vi "Rx Channel Section.vi"(8 "error in (no error)":errorcluster, 11 "Node Ptr":T1 format="%.0x") -> (0 "error out":errorcluster)   [LabVIEW 2019, in "UDP-Custom-Device System Explorer.lvlib"]
uses:
  UDP-Custom-Device System Explorer.lvlib
  <vilib>/NI VeriStand/Custom Device API/Custom Device Item Ref.ctl
  <vilib>/NI VeriStand/Custom Device API/Custom Device API.lvlib
panel:
  in  "Description":string
  out "Name":string
  in  "SHDocVw.IWebBrowser":refnum<k7>(container)
  in  "General Header":cluster{"Section Name":string}={"Section Name"="Receive Channels"}
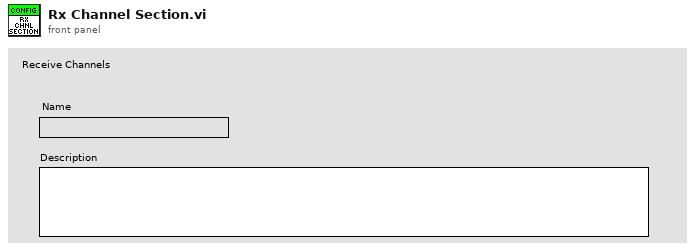
[diagram p1: front panel]
types:
  T1 = typedef "Custom Device API.lvlib/Custom Device Item Ref.ctl" = u64
  T2 = typedef "Custom Device API.lvlib/Custom Device Commands.ctl" = enum16{"Default", "Item renamed", "Shutdown", "Dynamic button pressed"}
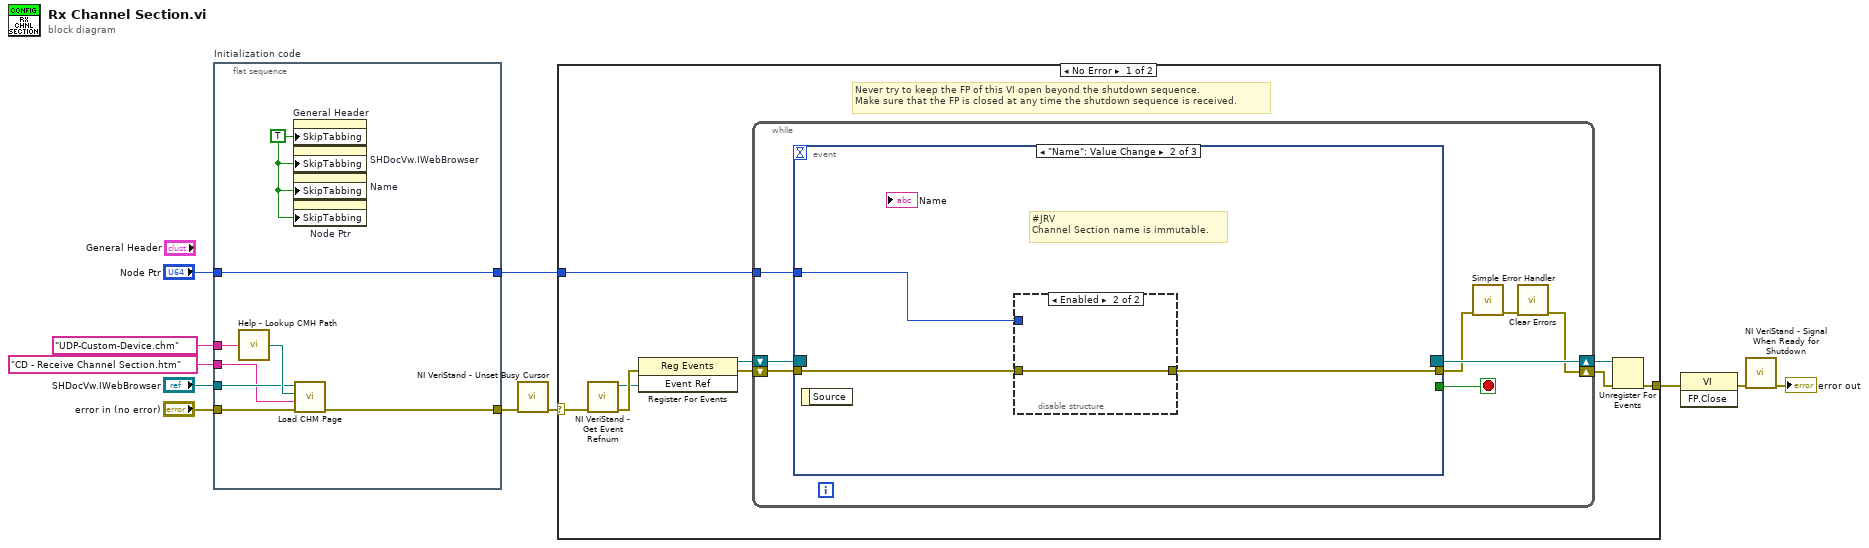
[diagram p0: block diagram]
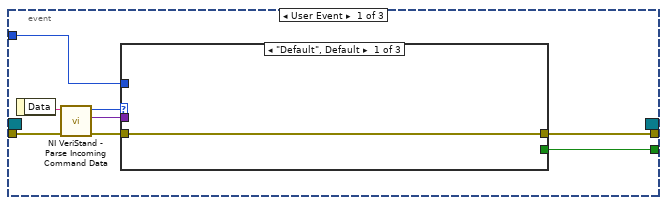
[diagram p2: hidden frame]
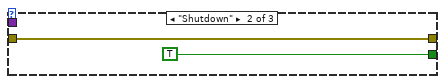
[diagram p3: hidden frame]
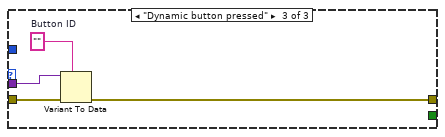
[diagram p4: hidden frame]
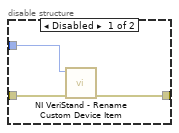
[diagram p5: hidden frame]
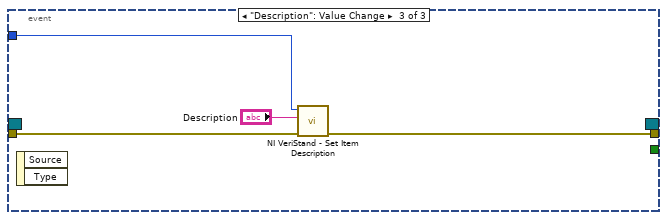
[diagram p6: hidden frame]
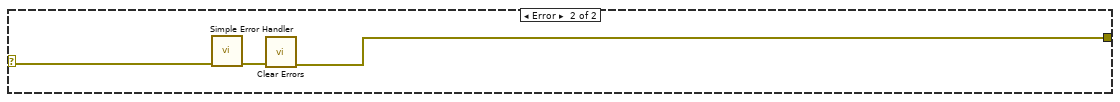
[diagram p7: hidden frame]
diagram:
  n1 = flat-sequence "Initialization code" {
    tunnel: "error in (no error)" -> [w18]
    tunnel: "Node Ptr" -> [w14]
    tunnel: [w13] -> w7
    tunnel: [w14] -> w4
    tunnel: "SHDocVw.IWebBrowser" -> [w17]
    tunnel: "CD - Receive Channel Section.htm" ("CD_CHM_Section") -> [w15]
    tunnel: "UDP-Custom-Device.chm" ("CD_CHM_FileName") -> [w16]
    frame #0 {
      w12 = TRUE ("Skip When Tabbing")
      n2 = call "Help - Lookup CMH Path.vi"("Main CMH File"=w16) -> ("Compiled CMH Path"=w19:path)
      n3 = property on="General Header" class="Clust (strict)"("SkipTabbing"=w12) -> ()  [unwired: 2 in, 2 out]
      n4 = property on="SHDocVw.IWebBrowser" class="AXCont"("SkipTabbing"=w12) -> ()  [unwired: 2 in, 2 out]
      n5 = property on="Name" class="Str"("SkipTabbing"=w12) -> ()  [unwired: 2 in, 2 out]
      n6 = property on="Node Ptr" class="DigNum (strict)"("SkipTabbing"=w12) -> ()  [unwired: 2 in, 2 out]
      n7 = call <vilib>:"Load CHM Page.vi"("error in (no error)"=w18, "HTML File"=w15, "Compiled CHM Path"=w19, "Web Browser Reference"=w17) -> ("error out"=w13:errorcluster)  [unwired: 7 in]
    }
  }
  n8 = call <vilib>:"NI VeriStand - Unset Busy Cursor.vi"("error in (no error)"=w7) -> ("error out"=w6:errorcluster)  [unwired: 10 out]
  n9 = case shown="No Error" w6 {
    selector: w6 -> [w20 w65]
    tunnel: [w25 w63] -> w11
    tunnel: w4 -> [w21 _]
    frame No Error {
      # "Never try to keep the FP of this VI open beyond the shutdown sequence.\nMake sure that the FP is closed at any time the shutdown sequence is received."
      n10 = call <vilib>:"NI VeriStand - Get Event Refnum.vi"("error in (no error)"=w20) -> ("error out"=w28:errorcluster, "Event Ref"=w24:refnum<user-event>)  [unwired: 9 out]
      n11 = register-events(error in=w28, w24) -> (reference out=w22:refnum<event-registration>, error out=w23:errorcluster)  [unwired: 1 in]
      n12 = while {
        tunnel: w21 -> [w32]
        shift-right: [w29] -> w26
        shift-left: w23 -> [w35]
        shift-right: [w36] -> w27
        shift-left: w22 -> [w34]
        stop <- w33 stop-if-true
        n13 = event shown="[1] \"Name\": Value Change" {
          selector: w34 -> [_ _ _]
          dyn-events: [_ _ _] -> w36
          timeout: _ -> [_ _ _]
          tunnel: w35 -> [w44 w54 w62]
          tunnel: [w40 _ _] -> w33
          tunnel: [w39 w52 w59] -> w31
          tunnel: w32 -> [w38 w53 w61]
          event User Event {
            n14 = event-data() -> ("Data"=w43:string)  [unwired: 1 out]
            n15 = call <vilib>:"NI VeriStand - Parse Incoming Command Data.vi"("error in (no error)"=w44, "Incoming data"=w43) -> ("error out"=w42:errorcluster, "Outgoing data"=w37:variant, "Action"=w41:T2)  [unwired: 7 out]
            n16 = case shown="\"Default\", Default" w41 {
              tunnel: w42 -> [w45 w46 w51]
              tunnel: [_ TRUE _] -> w40
              tunnel: [w45 w46 w48] -> w39
              tunnel: w38 -> [_ _ _]
              tunnel: w37 -> [_ _ w50]
              frame "Default", Default {
              }
              frame "Shutdown" {
              }
              frame "Dynamic button pressed" {
                w49 = ""  # Button ID
                n17 = Variant To Data(error in=w51, type=w49, Variant=w50) -> (error out=w48:errorcluster)  [unwired: 1 out]
              }
            }
          }
          event "Name": Value Change {
            # "#JRV\nChannel Section name is immutable."
            n18 = event-data() -> ()  [unwired: 2 out]
            n19 = disable-structure shown="Enabled" {
              disable-tunnel: w54 -> [w57 w58]
              disable-tunnel: w53 -> [w56 _]
              disable-tunnel: [w55 w58] -> w52
              frame Disabled {
                n20 = call <vilib>:"NI VeriStand - Rename Custom Device Item.vi"("error in (no error)"=w57, "Item Ref in"=w56) -> ("error out"=w55:errorcluster)  [unwired: 7 in, 2 out]
              }
              frame Enabled {
              }
            }
          }
          event "Description": Value Change {
            n21 = event-data() -> ()  [unwired: 3 out]
            n22 = call <vilib>:"NI VeriStand - Set Item Description.vi"("error in (no error)"=w62, "Description"="Description", "Item Ref in"=w61) -> ("error out"=w59:errorcluster)  [unwired: 6 in, 2 out]
          }
        }
        n23 = call <vilib>:"Simple Error Handler.vi"("error in (no error)"=w31) -> ("error out"=w30:errorcluster)  [unwired: 1 in, 7 out]
        n24 = call <vilib>:"Clear Errors.vi"("error in (no error)"=w30) -> ("error out"=w29:errorcluster)  [unwired: 1 in, 5 out]
      }
      n25 = Unregister For Events(event registration refnum=w27, error in=w26) -> (error out=w25:errorcluster)
    }
    frame Error {
      n26 = call <vilib>:"Simple Error Handler.vi"("error in (no error)"=w65) -> ("error out"=w64:errorcluster)  [unwired: 1 in, 7 out]
      n27 = call <vilib>:"Clear Errors.vi"("error in (no error)"=w64) -> ("error out"=w63:errorcluster)  [unwired: 1 in, 5 out]
    }
  }
  n28 = invoke class="VI" method="FP.Close"(error in=w11) -> (error out=w10:errorcluster)  [unwired: 2 in, 2 out]
  n29 = call <vilib>:"NI VeriStand - Signal When Ready for Shutdown.vi"("error in (no error)"=w10) -> ("error out"=→"error out":errorcluster)  [unwired: 10 out]
